vi "Helper Loop.vi"(8 "error in (no error)":errorcluster, 9 "Message Data":variant, 10 "Message":string, 11 "Helper Loop In":refnum<class "Helper Loop.lvclass">) -> (0 "error out":errorcluster, 3 "Helper Loop Out":refnum<class "Helper Loop.lvclass">)   [LabVIEW 2020, in "Helper Loop.lvclass"]
uses:
  Helper Loop.lvclass
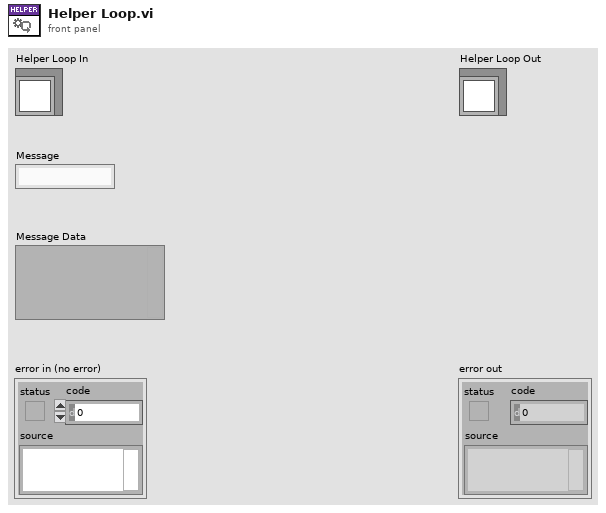
[diagram p1: front panel]
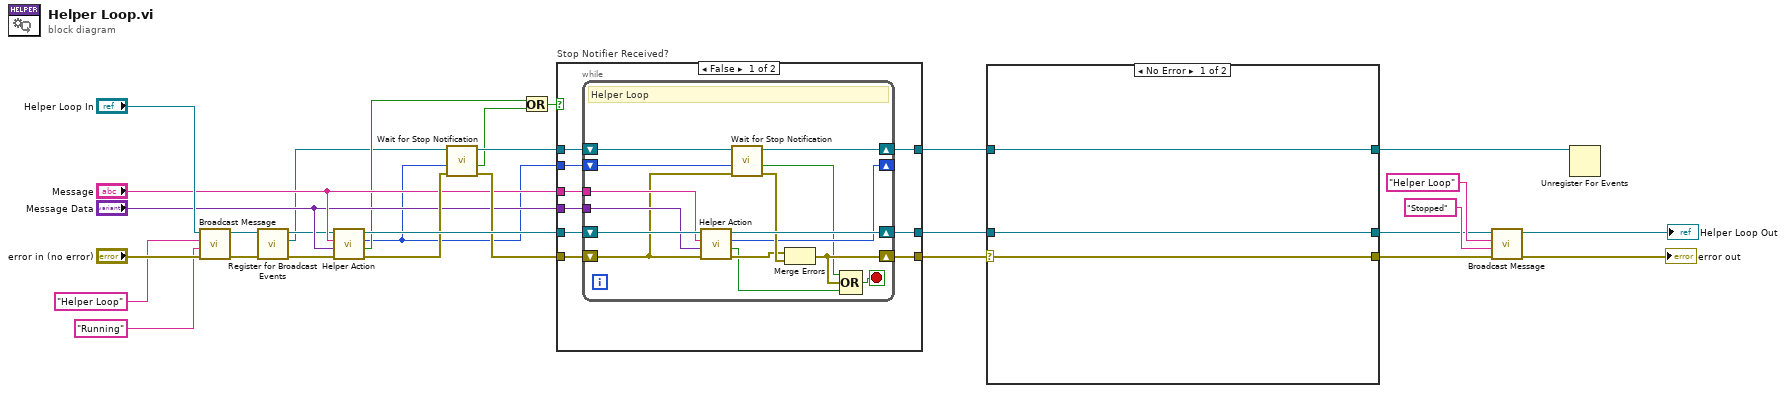
[diagram p0: block diagram]
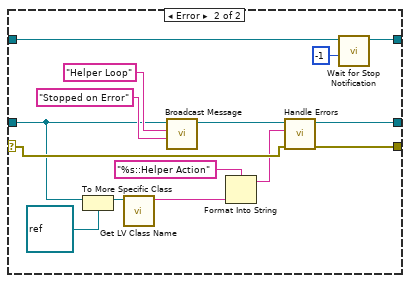
[diagram p3: hidden frame]
diagram:
  n1 = call-dynamic "Broadcast Message.vi"("error in (no error)"="error in (no error)", "Message Data"="Running" ("Message"), "Message"="Helper Loop", "Helper Loop in"="Helper Loop In") -> ("error out"=w13:errorcluster, "Helper Loop out"=w15:refnum<class "Helper Loop.lvclass">)  [unwired: 6 in]
  n2 = call "Register for Broadcast Events.vi"("error in (no error)"=w13, "Helper Loop in"=w15) -> ("error out"=w12:errorcluster, "Event Registration Refnum"=w11:refnum<event-registration>, "Helper Loop out"=w14:refnum<class "Helper Loop.lvclass">)  [unwired: 7 in]
  n3 = call-dynamic "Helper Action.vi"("error in (no error)"=w12, "Message Data"="Message Data", "Message"="Message", "Helper Loop In"=w14) -> ("error out"=w21:errorcluster, "Exit?"=w16:bool, "Loop Period [ms]"=w10:u32, "Helper Loop Out"=w23:refnum<class "Helper Loop.lvclass">)  [unwired: 4 in]
  n4 = call "Wait for Stop Notification.vi"("error in (no error)"=w21, "Loop Period [ms]"=w10, "Event Registration Refnum in"=w11) -> ("error out"=w20:errorcluster, "Stop Received?"=w9:bool, "Event Registration Refnum out"=w22:refnum<event-registration>)  [unwired: 6 in]
  n5 = Or(x=w16, y=w9) -> (x .or. y?=w17:bool)
  n6 = case "Stop Notifier Received?" shown="False" w17 {
    tunnel: [w38 w55] -> w25
    tunnel: [w37 w54] -> w24
    tunnel: [w36 w56] -> w8
    tunnel: w23 -> [w35 w55]
    tunnel: w22 -> [w34 w56]
    tunnel: w20 -> [w33 w54]
    tunnel: "Message" -> [w32 _]
    tunnel: "Message Data" -> [w31 _]
    tunnel: w10 -> [w30 _]
    frame False {
      n7 = while {
        shift-right: [w52] -> w38
        shift-left: w35 -> [w53]
        shift-right: [w44] -> w37
        shift-left: w33 -> [w41]
        tunnel: w32 -> [w49]
        tunnel: w31 -> [w48]
        shift-right: [w43] -> _
        shift-left: w30 -> [w46]
        shift-right: [w42] -> w36
        shift-left: w34 -> [w47]
        stop <- w51 stop-if-true
        # "Helper Loop"
        n8 = call-dynamic "Helper Action.vi"("error in (no error)"=w41, "Message Data"=w48, "Message"=w49, "Helper Loop In"=w53) -> ("error out"=w45:errorcluster, "Exit?"=w40:bool, "Loop Period [ms]"=w43:u32, "Helper Loop Out"=w52:refnum<class "Helper Loop.lvclass">)  [unwired: 4 in]
        n9 = call "Wait for Stop Notification.vi"("error in (no error)"=w41, "Loop Period [ms]"=w46, "Event Registration Refnum in"=w47) -> ("error out"=w50:errorcluster, "Stop Received?"=w39:bool, "Event Registration Refnum out"=w42:refnum<event-registration>)  [unwired: 6 in]
        n10 = Merge Errors(w45, w50) -> (w44:errorcluster)
        n11 = Compound Arithmetic op=OR(w39, w44, w40) -> (w51:bool)
      }
    }
    frame True {
    }
  }
  n12 = case shown="No Error" w24 {
    selector: w24 -> [w58 w71]
    tunnel: w25 -> [w59 w66]
    tunnel: [w59 w68] -> w4
    tunnel: [w58 w62] -> w1
    tunnel: w8 -> [w57 w63]
    tunnel: [w57 w60] -> w7
    frame No Error {
    }
    frame Error {
      n13 = To More Specific Class(target class=refnum<class> refnum ("object"), reference=w66) -> (specific class reference=w64:refnum<class>)  [unwired: 1 in, 1 out]
      n14 = call <vilib>:"Get LV Class Name.vi"("object"=w64) -> ("class name"=w69:string)  [unwired: 9 in, 1 out]
      n15 = call-dynamic "Broadcast Message.vi"("Message Data"="Stopped on Error" ("Description"), "Message"="Helper Loop", "Helper Loop in"=w66) -> ("Helper Loop out"=w72:refnum<class "Helper Loop.lvclass">)  [unwired: 7 in, 1 out]
      n16 = Format Into String(format string="%s::Helper Action", w69) -> (resulting string=w67:string)  [unwired: 2 in, 1 out]
      n17 = call-dynamic "Handle Errors.vi"("error in (no error)"=w71, "Location"=w67, "Helper Loop In"=w72) -> ("error out"=w62:errorcluster, "Helper Loop Out"=w68:refnum<class "Helper Loop.lvclass">)  [unwired: 7 in]
      n18 = call "Wait for Stop Notification.vi"("Loop Period [ms]"=-1, "Event Registration Refnum in"=w63) -> ("Event Registration Refnum out"=w60:refnum<event-registration>)  [unwired: 7 in, 2 out]
    }
  }
  n19 = call-dynamic "Broadcast Message.vi"("error in (no error)"=w1, "Message Data"="Stopped" ("Description"), "Message"="Helper Loop", "Helper Loop in"=w4) -> ("error out"=→"error out":errorcluster, "Helper Loop out"=→"Helper Loop Out":refnum<class "Helper Loop.lvclass">)  [unwired: 6 in]
  n20 = Unregister For Events(event registration refnum=w7) -> ()  [unwired: 1 in, 1 out]
